vi ".Net Symbol Information to G Symbol Information.vi"(0 "TwinCAT ADS in":refnum<class "TwinCAT ADS.lvclass">, 2 ".NET AdsSymbolInfo":refnum<k24>, 3 "error in (no error)":errorcluster) -> (7 "TwinCAT ADS out":refnum<class "TwinCAT ADS.lvclass">, 8 "Symbol Information":T1 {"Type ID" items=["ADST_VOID"=0, "ADST_INT16"=2, "ADST_INT32"=3, "ADST_REAL32"=4, "ADST_REAL64"=5, "ADST_INT8"=16, "ADST_UINT8"=17, "ADST_UINT16"=18, "ADST_UINT32"=19, "ADST_INT64"=20, "ADST_UINT64"=21, "ADST_STRING"=30, "ADST_WSTRING"=31, "ADST_REAL80"=32, "ADST_BIT"=33, "ADST_MAXTYPES"=34, "ADST_BIGTYPE"=65]; "Type Category" items=["Unknown, None"=0, "Primitive"=1, "Alias"=2, "Enum"=3, "Array"=4, "Struct"=5, "FunctionBlock"=6, "Program"=7, "Function"=8, "SubRange"=9, "String"=10, "Bitset"=12, "Pointer"=13, "Union"=14, "Reference"=15, "Interface"=16]}, 10 "error out":errorcluster)   [LabVIEW 2018, in "TwinCAT ADS.lvclass"]
uses:
  TwinCAT ADS.lvclass
  Controls/Symbol Information.ctl
  TwinCAT.Ads
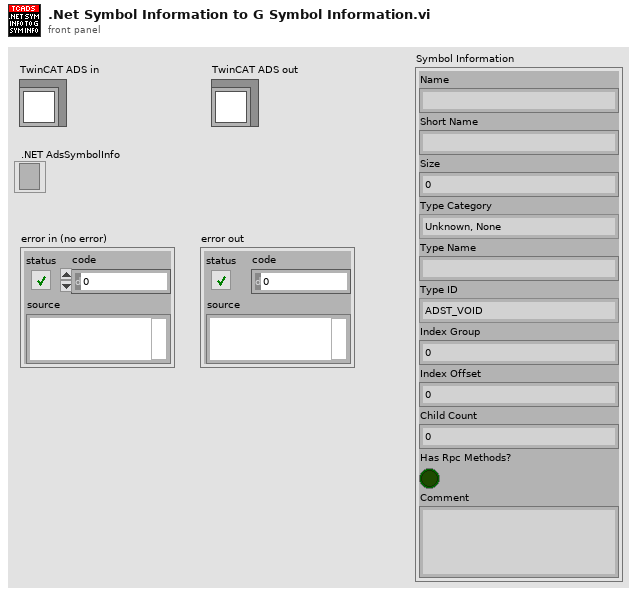
[diagram p1: front panel]
types:
  T1 = typedef "TwinCAT ADS.lvclass/Symbol Information.ctl" = cluster{"Name":string, "Short Name":string, "Size":i32, "Type Category":i32, "Type Name":string, "Type ID":i32, "Index Group":i64, "Index Offset":i64, "Child Count":i32, "Has Rpc Methods?":bool, "Comment":string}
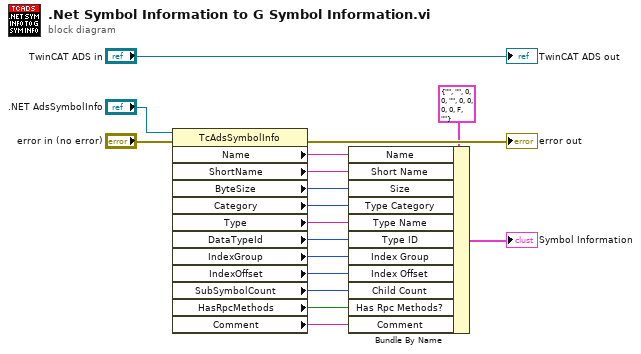
[diagram p0: block diagram]
diagram:
  n1 = property class="TcAdsSymbolInfo"(reference=".NET AdsSymbolInfo", error in="error in (no error)") -> (error out=→"error out":errorcluster, "Name"=w2:string, "ShortName"=w3:string, "ByteSize"=w4:i32, "Category"=w5:i32, "Type"=w6:string, "DataTypeId"=w7:i32, "IndexGroup"=w8:i64, "IndexOffset"=w9:i64, "SubSymbolCount"=w10:i32, "HasRpcMethods"=w11:bool, "Comment"=w12:string)  [unwired: 1 out]
  n2 = Bundle By Name(cluster=T1 {"Name"="", "Short Name"="", "Size"=0, "Type Category"=0, "Type Name"="", "Type ID"=0, "Index Group"=0, "Index Offset"=0, "Child Count"=0, "Has Rpc Methods?"=FALSE, "Comment"=""} ("Symbol Information"), "Name"=w2, "Short Name"=w3, "Size"=w4, "Type Category"=w5, "Type Name"=w6, "Type ID"=w7, "Index Group"=w8, "Index Offset"=w9, "Child Count"=w10, "Has Rpc Methods?"=w11, "Comment"=w12) -> (→"Symbol Information":T1)
  "TwinCAT ADS out" <- "TwinCAT ADS in"
